vi "BRig_Host__Loop_Consumer_RunState__typeTrial__subtypeStart_parse.vi"(11 "input_strCmd":string) -> (1 "output_LorR":u16, 2 "output_nTrial":u16, 3 "output_Start":bool)   [LabVIEW 2014]
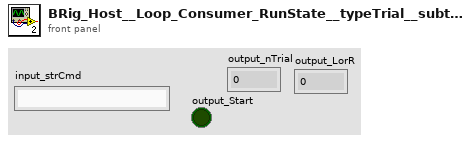
[diagram p1: front panel]
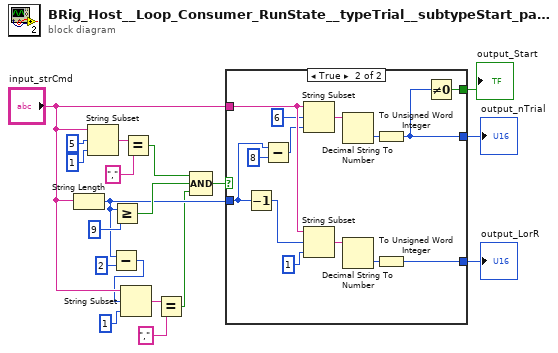
[diagram p0: block diagram]
diagram:
  n1 = String Length(string="input_strCmd") -> (length=w7:i32)
  n2 = String Subset(string="input_strCmd", offset (0)=5, length (rest)=1 ("offset (0)")) -> (substring=w17:string)
  n3 = Subtract(x=w7, y=2) -> (x-y=w5:i32)
  n4 = Greater Or Equal?(x=w7, y=9) -> (x >= y?=w14:bool)
  n5 = String Subset(string="input_strCmd", offset (0)=w5, length (rest)=1 ("offset (0)")) -> (substring=w9:string)
  n6 = Equal?(x=w17, y=",") -> (x = y?=w13:bool)
  n7 = Equal?(x=w9, y=",") -> (x = y?=w4:bool)
  n8 = Compound Arithmetic op=AND(w13, w14, w4) -> (w12:bool)
  n9 = case shown="True" w12 {
    tunnel: "input_strCmd" -> [_ w31]
    tunnel: w7 -> [_ w28]
    tunnel: [_ w21] -> w3
    tunnel: [_ w22] -> w2
    tunnel: [_ w20] -> w1
    frame False {
    }
    frame True {
      n10 = Decrement(x=w28) -> (x-1=w32:i32)
      n11 = Subtract(x=w28, y=8) -> (x-y=w27:i32)
      n12 = String Subset(string=w31, offset (0)=6, length (rest)=w27) -> (substring=w26:string)
      n13 = String Subset(string=w31, offset (0)=w32, length (rest)=1 ("offset (0)")) -> (substring=w25:string)
      n14 = Decimal String To Number(string=w26) -> (number=w24:i32)  [unwired: 2 in, 1 out]
      n15 = Decimal String To Number(string=w25) -> (number=w23:i32)  [unwired: 2 in, 1 out]
      n16 = To Unsigned Word Integer(number=w24) -> (unsigned 16bit integer=w21:u16)
      n17 = To Unsigned Word Integer(number=w23) -> (unsigned 16bit integer=w22:u16)
      n18 = Not Equal To 0?(x=w21) -> (x != 0?=w20:bool)
    }
  }
  "output_nTrial" <- w3
  "output_LorR" <- w2
  "output_Start" <- w1
